vi "WriteDataToFile.vi"(8 "error in (no error)":errorcluster, 11 "SettingsFile in":refnum<class "SettingsFile.lvclass">) -> (0 "error out":errorcluster, 2 "Path":path, 3 "SettingsFile out":refnum<class "SettingsFile.lvclass">)   [LabVIEW 2018, in "SettingsFile.lvclass"]
uses:
  SettingsFile.lvclass
  SettingsFile.lvclass/SettingsFile.ctl
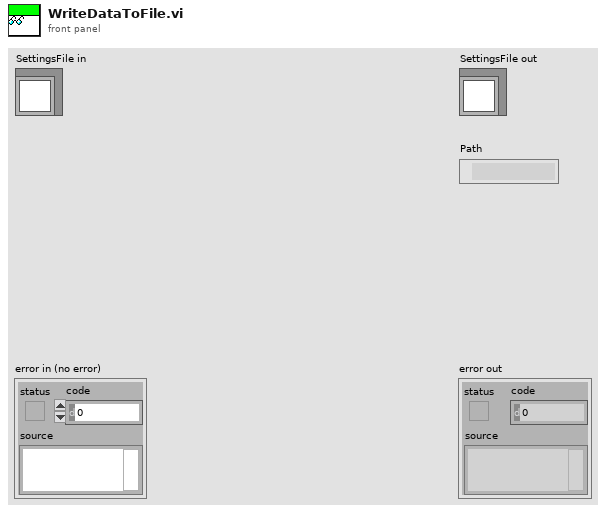
[diagram p1: front panel]
types:
  T1 = enum16{"open", "replace", "create", "open or create", "replace or create", "replace or create with confirmation"}
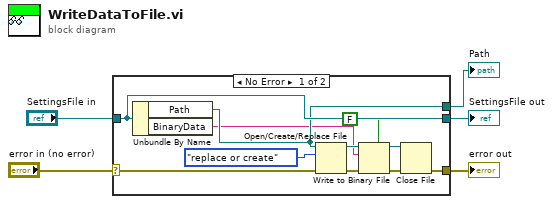
[diagram p0: block diagram]
diagram:
  n1 = case shown="No Error" "error in (no error)" {
    selector: "error in (no error)" -> [w10 w17]
    tunnel: [w7 w17] -> w4
    tunnel: [w16 w18] -> w2
    tunnel: "SettingsFile in" -> [w16 w18]
    tunnel: [w15 _] -> w1
    frame No Error {
      n2 = Unbundle By Name(w16) -> ("Path"=w15:path, "BinaryData"=w12:string)
      n3 = Open/Create/Replace File(file path (use dialog)=w15, error in=w10, operation (0:open)=T1."replace or create") -> (refnum out=w13:refnum<file>, error out=w11:errorcluster)  [unwired: 3 in, 1 out]
      n4 = Write to Binary File(file (use dialog)=w13, data=w12, error in=w11, 5:FALSE ("prepend array or string size? (T)")) -> (refnum out=w9:refnum<file>, error out=w8:errorcluster)  [unwired: 2 in, 1 out]
      n5 = Close File(refnum=w9, error in=w8) -> (error out=w7:errorcluster)  [unwired: 1 out]
    }
    frame Error {
    }
  }
  "error out" <- w4
  "SettingsFile out" <- w2
  "Path" <- w1
